vi "Get All VIs in Memory Including statically-referenced Reentrant Clones.vi"(8 "error in (no error)":errorcluster, 11 "App Refnum":refnum<vi>) -> (0 "error out":errorcluster, 2 "All VIs in Memory Including Reentrant Clones":string[](array[string]), 3 "App Refnum Out":refnum<vi>)   [LabVIEW 2011]
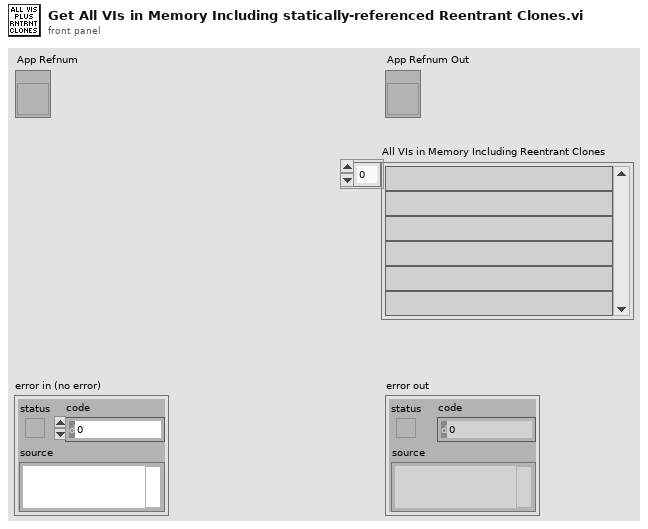
[diagram p1: front panel]
types:
  T1 = enum8{"Include the clone VI", "Include the original reentrant VI instead of the clone VI", "Include both the original reentrant VI and the clone VI"}
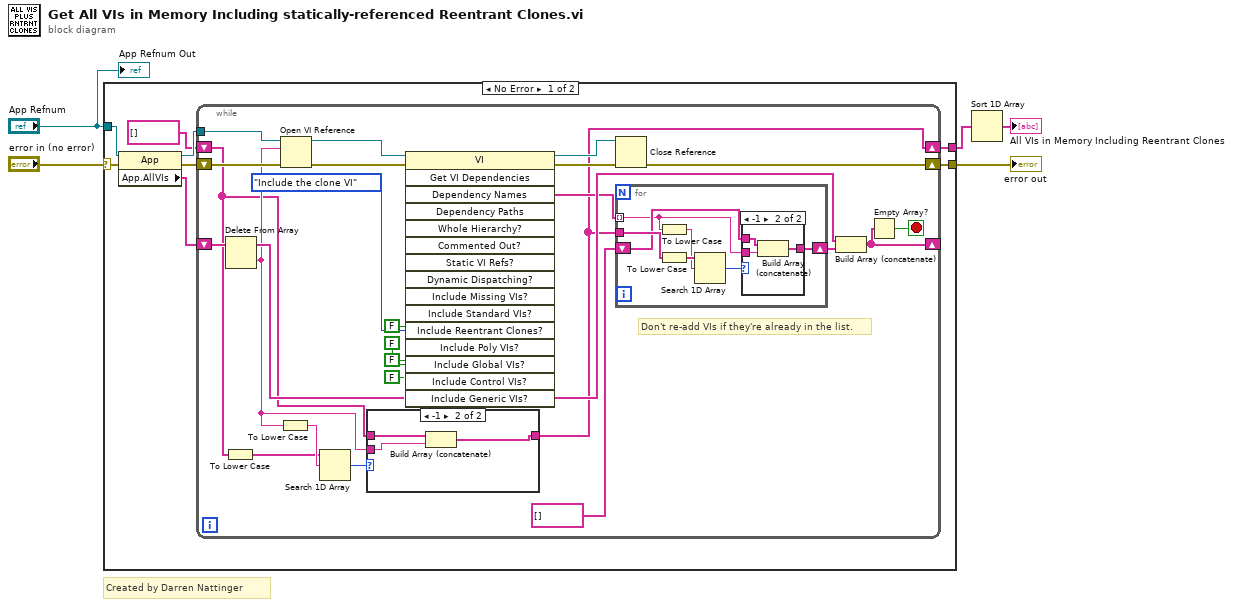
[diagram p0: block diagram]
diagram:
  # "Created by Darren Nattinger"
  n1 = case shown="No Error" "error in (no error)" {
    selector: "error in (no error)" -> [w13 w54]
    tunnel: [w7 w54] -> w4
    tunnel: "App Refnum" -> [w6 _]
    tunnel: [w8 _] -> w3
    frame No Error {
      n2 = property class="App"(reference=w6, error in=w13) -> (reference out=w11:refnum<vi>, error out=w12:errorcluster, "App.AllVIs"=w10:string[])
      n3 = while {
        tunnel: w11 -> [w37]
        shift-right: [w23] -> _
        shift-left: w10 -> [w35]
        shift-right: [w14] -> w8
        shift-left: string[] [] -> [w15]
        shift-right: [w25] -> w7
        shift-left: w12 -> [w38]
        stop <- w36 stop-if-true
        # "Don't re-add VIs if they're already in the list."
        n4 = To Lower Case(string=w15) -> (all lower case string=w18:string[])
        n5 = Delete From Array(array=w35) -> (deleted portion=w16:string, array with subset deleted=w24:string[])  [unwired: 2 in]
        n6 = To Lower Case(string=w16) -> (all lower case string=w19:string)
        n7 = Open VI Reference(application reference (local)=w37, vi path=w16, error in (no error)=w38) -> (vi reference=w34:refnum<vi>, error out=w33:errorcluster)  [unwired: 3 in]
        n8 = Search 1D Array(1D array=w18, element=w19) -> (index of element=w17:i32)  [unwired: 1 in]
        n9 = case shown="-1" w17 {
          tunnel: w15 -> [w39 w42]
          tunnel: w16 -> [_ w41]
          tunnel: [w39 w40] -> w14
          frame Default {
          }
          frame -1 {
            n10 = Build Array (concatenate)(w42, w41) -> (w40:string[])
          }
        }
        n11 = invoke class="VI" method="Get VI Dependencies"(reference=w34, error in=w33, "Include Reentrant Clones?"=T1."Include the clone VI", "Include Poly VIs?"=FALSE, "Include Global VIs?"=FALSE, "Include Control VIs?"=FALSE, "Include Generic VIs?"=FALSE) -> (reference out=w27:refnum<vi>, error out=w26:errorcluster, "Dependency Names"=w20:string[])  [unwired: 9 in, 13 out]
        n12 = Close Reference(reference=w27, error in (no error)=w26) -> (error out=w25:errorcluster)
        n13 = for {
          tunnel: w14 -> [w49]
          tunnel: w20 -> [w43] mode=indexing
          shift-right: [w44] -> w21
          shift-left: string[] [] -> [w45]
          n14 = To Lower Case(string=w43) -> (all lower case string=w47:string)
          n15 = To Lower Case(string=w49) -> (all lower case string=w48:string[])
          n16 = Search 1D Array(1D array=w48, element=w47) -> (index of element=w46:i32)  [unwired: 1 in]
          n17 = case shown="-1" w46 {
            tunnel: w45 -> [w50 w53]
            tunnel: [w50 w52] -> w44
            tunnel: w43 -> [_ w51]
            frame Default {
            }
            frame -1 {
              n18 = Build Array (concatenate)(w53, w51) -> (w52:string[])
            }
          }
        }
        n19 = Build Array (concatenate)(w24, w21) -> (w23:string[])
        n20 = Empty Array?(array=w23) -> (empty?=w36:bool)
      }
    }
    frame Error {
    }
  }
  "error out" <- w4
  n21 = Sort 1D Array(array=w3) -> (sorted array=→"All VIs in Memory Including Reentrant Clones":string[])
  "App Refnum Out" <- "App Refnum"
